vi "Calibration Image.vi"(2 "error in (no error)":errorcluster) -> (0 "error out":errorcluster, 1 "Calibration Image":T1)   [LabVIEW 2009, in "Camera.lvlib" / "Lens Distortion.lvlib"]
doc: "Creates a calibration image to use with remove lens distortion."
uses:
  Lens Distortion.lvlib
  <vilib>/vision/Image Controls.llb/IMAQ Image.ctl
  <vilib>/vision/NI_Vision_Development_Module.lvlib
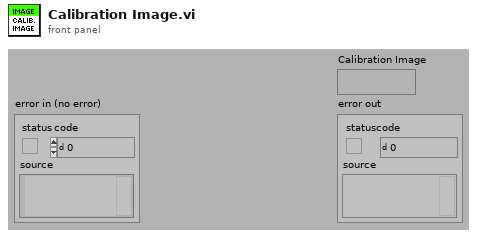
[diagram p1: front panel]
types:
  T1 = typedef "IMAQ Image.ctl" = refnum<image>
  T2 = cluster{"X Step":sgl, "Y Step":sgl, "Unit":u32, "Threshold Range":cluster{"Lower value":sgl, "Upper value":sgl}}
  T3 = cluster{"Distortion":u32, "Corrected Image Scaling":u32, "Corrected Image Learn ROI":u32, "Learn Error Map?":bool, "Learn Correction Table?":bool}
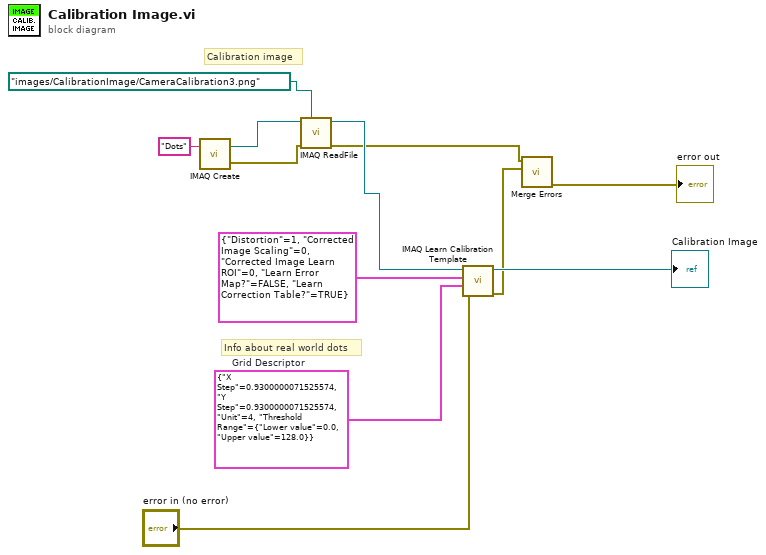
[diagram p0: block diagram]
diagram:
  w11 = T2 {"X Step"=0.93, "Y Step"=0.93, "Unit"=4, "Threshold Range"={"Lower value"=0.0, "Upper value"=128.0}}  # Grid Descriptor
  # "Calibration image"
  # "Info about real world dots"
  n1 = call "IMAQ Create"("Image Name"="Dots") -> ("New Image"=w8:T1, "error out"=w5:errorcluster)  [unwired: 4 in]
  n2 = call "IMAQ ReadFile"("File Path"=path "images/CalibrationImage/CameraCalibration3.png" ("base path"), "error in (no error)"=w5, "Image"=w8) -> ("error out"=w4:errorcluster, "Image Out"=w6:T1)  [unwired: 4 in, 3 out]
  n3 = call "IMAQ Learn Calibration Template"("error in (no error)"="error in (no error)", "Grid Descriptor"=w11, "Calibration Learn Setup"=T3 {"Distortion"=1, "Corrected Image Scaling"=0, "Corrected Image Learn ROI"=0, "Learn Error Map?"=FALSE, "Learn Correction Table?"=TRUE}, "Image"=w6) -> ("error out"=w3:errorcluster, "Calibrated Image"=→"Calibration Image":T1)  [unwired: 5 in, 1 out]
  n4 = call <vilib>:"Merge Errors.vi"("error in 2 (no error)"=w3, "error in 1 (no error)"=w4) -> ("error out"=→"error out":errorcluster)  [unwired: 5 in]
